vi "Initilaize Views.vi"(8 "error in (no error)":errorcluster, 11 "Example Controller in":refnum<class "Example Controller Actor.lvclass">) -> (0 "error out":errorcluster, 3 "Example Controller out":refnum<class "Example Controller Actor.lvclass">)   [LabVIEW 2017, in "Example GUI View Actor.lvlib" / "Example Controller Actor.lvclass"]
uses:
  Example Controller Actor.lvclass
  C:/Projects/Shared Libraries/Event Actors/Controller Actor/Controller Actor.lvclass
  Example GUI Container/Example GUI Container.lvclass
  C:/Projects/Shared Libraries/Event Actors/View Actor/View Actor.lvclass
  View Actor/View Actor.lvclass/View Actor.ctl
  Example Controller Actor.lvclass/Example Controller Actor.ctl
  View Actor/properties/Write Name.vi
  Example Controller Actor/Example Controller Actor/Example Controller Actor.lvclass
  Controller Actor/Controller Actor.lvclass
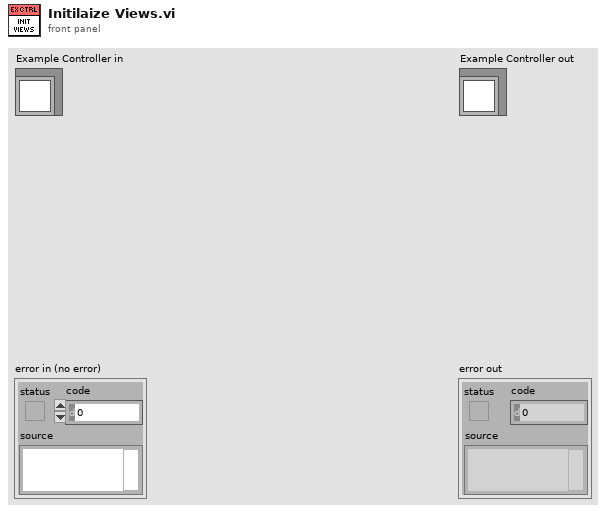
[diagram p1: front panel]
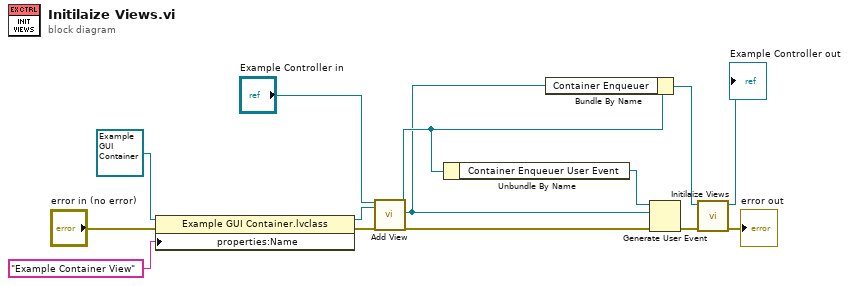
[diagram p0: block diagram]
diagram:
  n1 = property class="Example GUI Container.lvclass"(reference=refnum<class "Example GUI Container.lvclass"> refnum ("Example GUI View Actor.lvlib:Example GUI Container.lvclass"), error in="error in (no error)", "properties:Name"="Example Container View" ("Debug Alias")) -> (reference out=w12:refnum<class "Example GUI Container.lvclass">, error out=w10:errorcluster)
  n2 = call "Add View.vi"("Controller Actor in"="Example Controller in", "View Actor"=w12, "error in (no error)"=w10) -> ("Controller Actor out"=w3:refnum<class "Example Controller Actor.lvclass">, "View Enqueuer"=w1:refnum<class "Message Enqueuer.lvclass">, "error out"=w6:errorcluster)  [unwired: 14 in]
  n3 = Unbundle By Name(w3) -> ("Container Enqueuer User Event"=w2:refnum<user-event>)
  n4 = Bundle By Name(cluster=w3, "Container Enqueuer"=w1) -> (w5:refnum<class "Example Controller Actor.lvclass">)
  n5 = Generate User Event(user event=w2, event data cluster=w1, error in=w6) -> (error out=w4:errorcluster)  [unwired: 1 in, 1 out]
  n6 = call-parent "Initilaize Views.vi"("error in (no error)"=w4, "Example Controller in"=w5) -> ("error out"=→"error out":errorcluster, "Example Controller out"=→"Example Controller out":refnum<class "Example Controller Actor.lvclass">)  [unwired: 8 in]
